vi "CRYPlot Intensity Graph.vi"(6 "Graph Set?":bool, 7 "pGraph VI In":refnum<vi>, 9 "Flattened Intensity Property":string, 11 "Selected Rows In":i32[](array[numeric])) -> (0 "ItemSyms":i32[](array[numeric]), 1 "Color Info":u32[](array[numeric]), 2 "Wave Names":string[](array[string]), 3 "All Rows Out":i32[](array[numeric]))   [LabVIEW 2013]
uses:
  <vilib>/Analysis/4window.llb/windowTd.ctl
  CRYWindow/DataView/Control/CRYIntensity Property.ctl
  <vilib>/Analysis/NI_AALPro.lvlib
panel:
  in  "Intensity Property":T1 {"Type" items=["Rectangle"=0, "Hanning"=1, "Hamming"=2, "Blackman-Harris"=3, "Exact Blackman"=4, "Blackman"=5, "Flat Top"=6, "4 Term B-Harris"=7, "7 Term B-Harris"=8, "Low Sidelobe"=9, "Blackman Nuttall"=11, "Triangle"=30, "Bartlett-Hanning"=31, "Bohman"=32, "Parzen"=33, "Welch"=34, "Kaiser"=60, "Dolph-Chebyshev"=61, "Gaussian"=62]}
  in  "32 ice":u32[](array[numeric])=[2155776, 2155776, 2155776, 2155776, 2155776, 2155776, 2155776, 2155776, 127491, 127491, 127491, 127491, 127491, 127491, 127491, 127491, 522752, 522752, 522752, 522752, 522752, 522752, 522752, 522752, 64018, 64018, 64018, 64018, 64018, 64018, 64018, 64018, 63778, 63778, 63778, 63778, 63778, 63778, 63778, 63778, 63790, 63790, 63790, 63790, 63790, 63790, 63790, 63790, 63797, 63797, 63797, 63797, 63797, 63797, 63797, 63797, 63807, 63807, 63807, 63807, 63807, 63807, 63807, 63807, 64068, 64068, 64068, 64068, 64068, 64068, 64068, 64068, 63828, 63828, 63828, 63828, 63828, 63828, 63828, 63828, 63833, 63833, 63833, 63833, 63833, 63833, 63833, 63833, 63836, 63836, 63836, 63836, 63836, 63836, 63836, 63836, 63836, 63836, 63836, 63836, 63836, 63836, 63836, 63836, 61790, 61790, 61790, 61790, 61790, 61790, 61790, 61790, 58464, 58464, 58464, 58464, 58464, 58464, 58464, 58464, 55387, 55387, 55387, 55387, 55387, 55387, 55387, 55387, 51286, 51286, 51286, 51286, 51286, 51286, 51286, 51286, 47440, 47440, 47440, 47440, 47440, 47440, 47440, 47440, 40284, 40284, 40284, 40284, 40284, 40284, 40284, 40284, 34154, 34154, 34154, 34154, 34154, 34154, 34154, 34154, 28540, 28540, 28540, 28540, 28540, 28540, 28540, 28540, 20113, 20113, 20113, 20113, 20113, 20113, 20113, 20113, 12193, 12193, 12193, 12193, 12193, 12193, 12193, 12193, 12714, 12714, 12714, 12714, 12714, 12714, 12714, 12714, 7351, 7351, 7351, 7351, 7351, 7351, 7351, 7351, 4800, 4800, 4800, 4800, 4800, 4800, 4800, 4800, 195, 195, 195, 195, 195, 195, 195, 195, 189, 189, 189, 189, 189, 189, 189, 189, 183, 183, 183, 183, 183, 183, 183, 183, 175, 175, 175, 175, 175, 175, 175, 175, 164, 164, 164, 164, 164, 164, 164, 164, 155, 155, 155, 155, 155, 155, 155, 155]
  in  "32 colour":u32[](array[numeric])=[2161664, 2161664, 2161664, 2161664, 2161664, 2161664, 2161664, 2161664, 588800, 588800, 588800, 588800, 588800, 588800, 588800, 588800, 523264, 523264, 523264, 523264, 523264, 523264, 523264, 523264, 64512, 64512, 64512, 64512, 64512, 64512, 64512, 64512, 64512, 64512, 64512, 64512, 64512, 64512, 64512, 64512, 64512, 64512, 64512, 64512, 64512, 64512, 64512, 64512, 64512, 64512, 64512, 64512, 64512, 64512, 64512, 64512, 64512, 64512, 64512, 64512, 64512, 64512, 64512, 64512, 64512, 64512, 64512, 64512, 64512, 64512, 64512, 64512, 64512, 64512, 64512, 64512, 64512, 64512, 64512, 64512, 64512, 64512, 64512, 64512, 64512, 64512, 64512, 64512, 64512, 64512, 64512, 64512, 64512, 64512, 64512, 64512, 64512, 64512, 64512, 64512, 64512, 64512, 64512, 64512, 64512, 64512, 64512, 64512, 64512, 64512, 64512, 64512, 64512, 64512, 64512, 64512, 64512, 64512, 64512, 64512, 64512, 64512, 64512, 64512, 64512, 64512, 64512, 64512, 64525, 64525, 64525, 64525, 64525, 64525, 64525, 64525, 64541, 64541, 64541, 64541, 64541, 64541, 64541, 64541, 64557, 64557, 64557, 64557, 64557, 64557, 64557, 64557, 64573, 64573, 64573, 64573, 64573, 64573, 64573, 64573, 64333, 64333, 64333, 64333, 64333, 64333, 64333, 64333, 64349, 64349, 64349, 64349, 64349, 64349, 64349, 64349, 64621, 64621, 64621, 64621, 64621, 64621, 64621, 64621, 64636, 64636, 64636, 64636, 64636, 64636, 64636, 64636, 64653, 64653, 64653, 64653, 64653, 64653, 64653, 64653, 64670, 64670, 64670, 64670, 64670, 64670, 64670, 64670, 64685, 64685, 64685, 64685, 64685, 64685, 64685, 64685, 64701, 64701, 64701, 64701, 64701, 64701, 64701, 64701, 64717, 64717, 64717, 64717, 64717, 64717, 64717, 64717, 64733, 64733, 64733, 64733, 64733, 64733, 64733, 64733, 64749, 64749, 64749, 64749, 64749, 64749, 64749, 64749, 64764, 64764, 64764, 64764, 64764, 64764, 64764, 64764]
  in  "256 log down":u32[](array[numeric])=[16777215, 14737632, 13487565, 12632256, 11908533, 11382189, 10921638, 10526880, 10132122, 9803157, 9539985, 9276813, 9013641, 8816262, 8553090, 8421504, 8224125, 8026746, 7895160, 7697781, 7566195, 7434609, 7303023, 7171437, 7039851, 6908265, 6776679, 6710886, 6579300, 6447714, 6381921, 6316128, 6184542, 6118749, 5987163, 5921370, 5855577, 5789784, 5658198, 5592405, 5526612, 5460819, 5395026, 5329233, 5263440, 5197647, 5131854, 5066061, 5000268, 4934475, 4868682, 4802889, 4737096, 4671303, 4605510, 4605510, 4539717, 4473924, 4408131, 4342338, 4342338, 4276545, 4210752, 4210752, 4144959, 4079166, 4013373, 4013373, 3947580, 3881787, 3881787, 3815994, 3750201, 3750201, 3684408, 3684408, 3618615, 3552822, 3552822, 3487029, 3487029, 3421236, 3421236, 3355443, 3289650, 3289650, 3223857, 3223857, 3158064, 3158064, 3092271, 3092271, 3026478, 3026478, 2960685, 2960685, 2894892, 2894892, 2829099, 2829099, 2763306, 2763306, 2763306, 2697513, 2697513, 2631720, 2631720, 2565927, 2565927, 2500134, 2500134, 2500134, 2434341, 2434341, 2368548, 2368548, 2368548, 2302755, 2302755, 2236962, 2236962, 2236962, 2171169, 2171169, 2171169, 2105376, 2105376, 2105376, 2039583, 2039583, 1973790, 1973790, 1973790, 1907997, 1907997, 1907997, 1842204, 1842204, 1842204, 1776411, 1776411, 1776411, 1710618, 1710618, 1710618, 1644825, 1644825, 1644825, 1579032, 1579032, 1579032, 1579032, 1513239, 1513239, 1513239, 1447446, 1447446, 1447446, 1381653, 1381653, 1381653, 1381653, 1315860, 1315860, 1315860, 1315860, 1250067, 1250067, 1250067, 1184274, 1184274, 1184274, 1184274, 1118481, 1118481, 1118481, 1118481, 1052688, 1052688, 1052688, 1052688, 986895, 986895, 986895, 921102, 921102, 921102, 921102, 921102, 855309, 855309, 855309, 855309, 789516, 789516, 789516, 789516, 723723, 723723, 723723, 723723, 657930, 657930, 657930, 657930, 657930, 592137, 592137, 592137, 592137, 526344, 526344, 526344, 526344, 526344, 460551, 460551, 460551, 460551, 460551, 394758, 394758, 394758, 394758, 328965, 328965, 328965, 328965, 328965, 263172, 263172, 263172, 263172, 263172, 197379, 197379, 197379, 197379, 197379, 131586, 131586, 131586, 131586, 131586, 131586, 65793, 65793, 65793, 65793, 65793, 0, 0, 0, 0, 0, 0]
  in  "256 log up":u32[](array[numeric])=[16777215, 16777215, 16777215, 16777215, 16777215, 16777215, 16711422, 16711422, 16711422, 16711422, 16711422, 16645629, 16645629, 16645629, 16645629, 16645629, 16645629, 16579836, 16579836, 16579836, 16579836, 16579836, 16514043, 16514043, 16514043, 16514043, 16514043, 16448250, 16448250, 16448250, 16448250, 16448250, 16316664, 16382457, 16382457, 16382457, 16382457, 16316664, 16316664, 16316664, 16316664, 16250871, 16250871, 16250871, 16250871, 16250871, 16185078, 16185078, 16185078, 16185078, 16119285, 16119285, 16119285, 16119285, 16119285, 16053492, 16053492, 16053492, 16053492, 15987699, 15987699, 15987699, 15987699, 15921906, 15987699, 15921906, 15921906, 15856113, 15856113, 15856113, 15856113, 15856113, 15790320, 15790320, 15790320, 15724527, 15724527, 15724527, 15724527, 15658734, 15658734, 15658734, 15658734, 15592941, 15592941, 15592941, 15592941, 15527148, 15527148, 15527148, 15461355, 15461355, 15461355, 15461355, 15395562, 15395562, 15395562, 15395562, 15329769, 15329769, 15329769, 15263976, 15263976, 15263976, 15198183, 15198183, 15198183, 15198183, 15132390, 15132390, 15132390, 15066597, 15066597, 15066597, 15000804, 15000804, 15000804, 14935011, 14935011, 14935011, 14869218, 14869218, 14869218, 14803425, 14803425, 14803425, 14737632, 14737632, 14671839, 14671839, 14671839, 14606046, 14606046, 14606046, 14540253, 14540253, 14540253, 14474460, 14474460, 14408667, 14408667, 14408667, 14342874, 14342874, 14277081, 14277081, 14277081, 14211288, 14211288, 14145495, 14145495, 14079702, 14079702, 14013909, 14013909, 14013909, 13948116, 13948116, 13882323, 13882323, 13816530, 13816530, 13750737, 13750737, 13684944, 13684944, 13619151, 13619151, 13553358, 13553358, 13487565, 13487565, 13421772, 13421772, 13355979, 13290186, 13290186, 13224393, 13224393, 13158600, 13092807, 13092807, 13027014, 13027014, 12961221, 12895428, 12895428, 12829635, 12763842, 12763842, 12698049, 12632256, 12566463, 12566463, 12500670, 12434877, 12434877, 12369084, 12303291, 12237498, 12171705, 12171705, 12105912, 12040119, 11974326, 11908533, 11842740, 11776947, 11711154, 11645361, 11579568, 11513775, 11447982, 11382189, 11316396, 11250603, 11184810, 11119017, 10987431, 10921638, 10855845, 10790052, 10658466, 10592673, 10461087, 10395294, 10329501, 10197915, 10066329, 10000536, 9868950, 9737364, 9605778, 9474192, 9342606, 9211020, 9079434, 8882055, 8750469, 8553090, 8421504, 8224125, 7960953, 7763574, 7500402, 7237230, 6974058, 6645093, 6316128, 5855577, 5395026, 4868682, 4210752, 3289650, 2105376, 0]
  in  "256 fire":u32[](array[numeric])=[16777215, 16777215, 16777215, 16777215, 16777215, 16777215, 16777215, 16777215, 16777212, 16777209, 16777205, 16777202, 16777199, 16777196, 16777193, 16777190, 16777186, 16777183, 16777180, 16777177, 16777174, 16777170, 16777167, 16777164, 16777161, 16777158, 16777154, 16777151, 16777148, 16777145, 16777142, 16777139, 16777135, 16777132, 16777129, 16777126, 16777123, 16777119, 16777116, 16777113, 16777110, 16777107, 16777103, 16777100, 16777097, 16777094, 16777091, 16777088, 16777084, 16777081, 16777078, 16777075, 16777072, 16777068, 16777065, 16777062, 16777059, 16777056, 16777052, 16777049, 16777046, 16777043, 16777040, 16777037, 16777033, 16777030, 16777027, 16777024, 16777021, 16777017, 16777014, 16777011, 16777008, 16777005, 16777001, 16776998, 16776995, 16776992, 16776989, 16776986, 16776982, 16776979, 16776976, 16776973, 16776970, 16776966, 16776963, 16776960, 16776192, 16775424, 16774400, 16773632, 16772864, 16772096, 16771328, 16770560, 16769536, 16768768, 16768000, 16767232, 16766464, 16765440, 16764672, 16763904, 16763136, 16762368, 16761344, 16760576, 16759808, 16759040, 16758272, 16757504, 16756480, 16755712, 16754944, 16754176, 16753408, 16752384, 16751616, 16750848, 16750080, 16749312, 16748288, 16747520, 16746752, 16745984, 16745216, 16744448, 16743424, 16742656, 16741888, 16741120, 16740352, 16739328, 16738560, 16737792, 16737024, 16736256, 16735232, 16734464, 16733696, 16732928, 16732160, 16731392, 16730368, 16729600, 16728832, 16728064, 16727296, 16726272, 16725504, 16724736, 16723968, 16723200, 16722176, 16721408, 16720640, 16719872, 16719104, 16718336, 16717312, 16716544, 16715776, 16715008, 16714240, 16713216, 16712448, 16711680, 16515072, 16318464, 16056320, 15859712, 15663104, 15466496, 15269888, 15073280, 14811136, 14614528, 14417920, 14221312, 14024704, 13762560, 13565952, 13369344, 13172736, 12976128, 12713984, 12517376, 12320768, 12124160, 11927552, 11730944, 11468800, 11272192, 11075584, 10878976, 10682368, 10420224, 10223616, 10027008, 9830400, 9633792, 9371648, 9175040, 8978432, 8781824, 8585216, 8388608, 8126464, 7929856, 7733248, 7536640, 7340032, 7077888, 6881280, 6684672, 6488064, 6291456, 6029312, 5832704, 5636096, 5439488, 5242880, 5046272, 4784128, 4587520, 4390912, 4194304, 3997696, 3735552, 3538944, 3342336, 3145728, 2949120, 2686976, 2490368, 2293760, 2097152, 1900544, 1703936, 1441792, 1245184, 1048576, 851968, 655360, 393216, 196608, 65793, 65793, 65793, 65793, 65793, 65793, 65793, 65793, 0]
  in  "window info":cluster{"type":T2, "length":i32}={"type"=1, "length"=64} {"type" items=["Rectangle"=0, "Hanning"=1, "Hamming"=2, "Blackman-Harris"=3, "Exact Blackman"=4, "Blackman"=5, "Flat Top"=6, "4 Term B-Harris "=7, "7 Term B-Harris"=8, "Low Sidelobe"=9, "Blackman Nuttall"=11, "Triangle"=30, "Bartlett-Hanning"=31, "Bohman"=32, "Parzen"=33, "Welch"=34, "Kaiser"=60, "Dolph-Chebyshev"=61, "Gaussian"=62]}
  in  "time-freq sampling info":cluster{"time steps":i32, "frequency bins":i32}={"time steps"=512, "frequency bins"=1024}
  in  "256 rainbow":u32[](array[numeric])=[16777215, 8126719, 7864574, 7536895, 7274750, 6947071, 6684926, 6357247, 6095102, 5767423, 5505278, 5177599, 4915454, 4587775, 4325630, 3997951, 3735806, 3408127, 3145982, 2818303, 2556158, 2228479, 1966334, 1638655, 1376510, 1048831, 786686, 459007, 196862, 767, 1790, 3071, 4094, 5375, 6398, 7679, 8702, 9983, 11006, 12287, 13310, 14591, 15614, 16895, 17918, 19199, 20222, 21503, 22526, 23807, 24830, 26111, 27134, 28415, 29438, 30719, 31486, 33023, 33790, 35327, 36094, 37631, 38398, 39935, 40702, 42239, 43006, 44543, 45310, 46847, 47614, 49151, 49918, 51455, 52222, 53759, 54526, 56063, 56830, 58367, 59134, 60671, 61694, 62975, 63998, 65279, 65274, 65527, 65265, 65518, 65256, 65509, 65247, 65500, 65238, 65491, 65229, 65482, 65220, 65473, 65211, 65464, 65202, 65455, 65193, 65446, 65184, 65437, 65175, 65428, 65166, 65419, 65157, 65410, 65149, 65401, 65140, 65392, 65131, 65383, 65122, 65374, 65113, 65365, 65104, 65356, 65095, 65347, 65086, 65338, 65077, 65329, 65068, 65320, 65059, 65311, 65050, 65302, 65041, 65293, 65032, 65284, 130560, 392960, 720384, 982784, 1310208, 1572608, 1900032, 2162432, 2489856, 2752256, 3079680, 3342080, 3669504, 3931904, 4259328, 4521728, 4849152, 5111552, 5438976, 5701376, 6028800, 6291200, 6618624, 6881024, 7208448, 7470848, 7798272, 8126208, 8322560, 8716032, 8912384, 9305856, 9502208, 9895680, 10092032, 10485504, 10681856, 11075328, 11271680, 11665152, 11861504, 12254976, 12451328, 12844800, 13041152, 13434624, 13630976, 14024448, 14220800, 14614272, 14810624, 15204096, 15400448, 15793920, 15990272, 16383744, 16580096, 16776192, 16709376, 16773888, 16707072, 16771584, 16704768, 16769280, 16702464, 16766976, 16700160, 16764672, 16697856, 16762368, 16695552, 16760064, 16693248, 16757760, 16690944, 16755456, 16688640, 16753152, 16686336, 16750848, 16684032, 16748544, 16681728, 16746240, 16679680, 16743936, 16677376, 16741632, 16675072, 16739328, 16672768, 16737024, 16670464, 16734720, 16668160, 16732416, 16665856, 16730112, 16663552, 16727808, 16661248, 16725504, 16658944, 16723200, 16656640, 16720896, 16654336, 16718592, 16652032, 16716288, 16649728, 16713984, 16712960, 0]
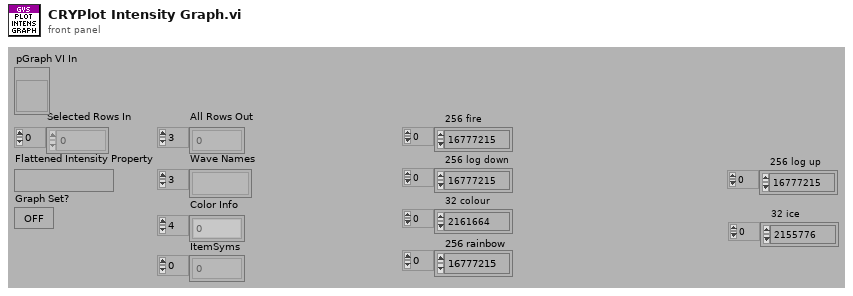
[diagram p1: front panel]
types:
  T1 = typedef "CRYIntensity Property.ctl" = cluster{"Time Steps":i32, "Frequency Bins":i32, "Type":u32, "Length":i32, "Map Type":enum16{"fire", "rainbow", "grey", "inverse grey", "ice", "original"}}
  T2 = typedef "NI_AALPro.lvlib/windowTd.ctl" = u32
  T3 = typedef "CRYWaveform Cluster.ctl" = cluster{"Waveform":cluster{"X0":dbl, "dX":dbl, "Y":sgl[]}, "X data":u16, "Y data":u16, "Y axis":u16, "X unit":string, "Y unit":string, "Y dB ref":dbl, "display Y":bool, "display X":bool, "Overload?":bool, "Test Info":string, "Step No.":i32, "Name":string, "protected":bool, "Sqc history":string[], "Signal Channel ID":i32, "Plot Settings":cluster{"Color":u32, "Interpolation":u8, "Point Style":u8, "Line Style":u8, "Point Color":u32, "Line Width":u8, "Bar Plot Style":u8, "Fill To":i16}, "AutoProtect":bool}
  T4 = enum16{"OK", "Yes", "YesNo", "YesNoCancel", "ReplaceAppend"}
  T5 = typedef "CRYStimulus Test Infor Cluster.ctl" = cluster{"Stimulus Type":string, "Signal Type":string, "In/Out":bool, "FAPS":cluster{"freq":dbl, "ampl":dbl, "cycles":dbl, "samples":i32}[], "Sampling Rate":dbl, "Samples":i32, "Analysis Param":string, "Resolution":u16, "Steps":u32, "Analysis Value":dbl[], "Diff Freq":dbl, "FStart":dbl, "FStop":dbl, "Calibration Param":string, "Anti Alias":dbl, "Level Out1":dbl, "Level Out2":dbl, "EQ":bool}
  T6 = enum16{"fire", "rainbow", "grey", "inverse grey", "ice", "original"}
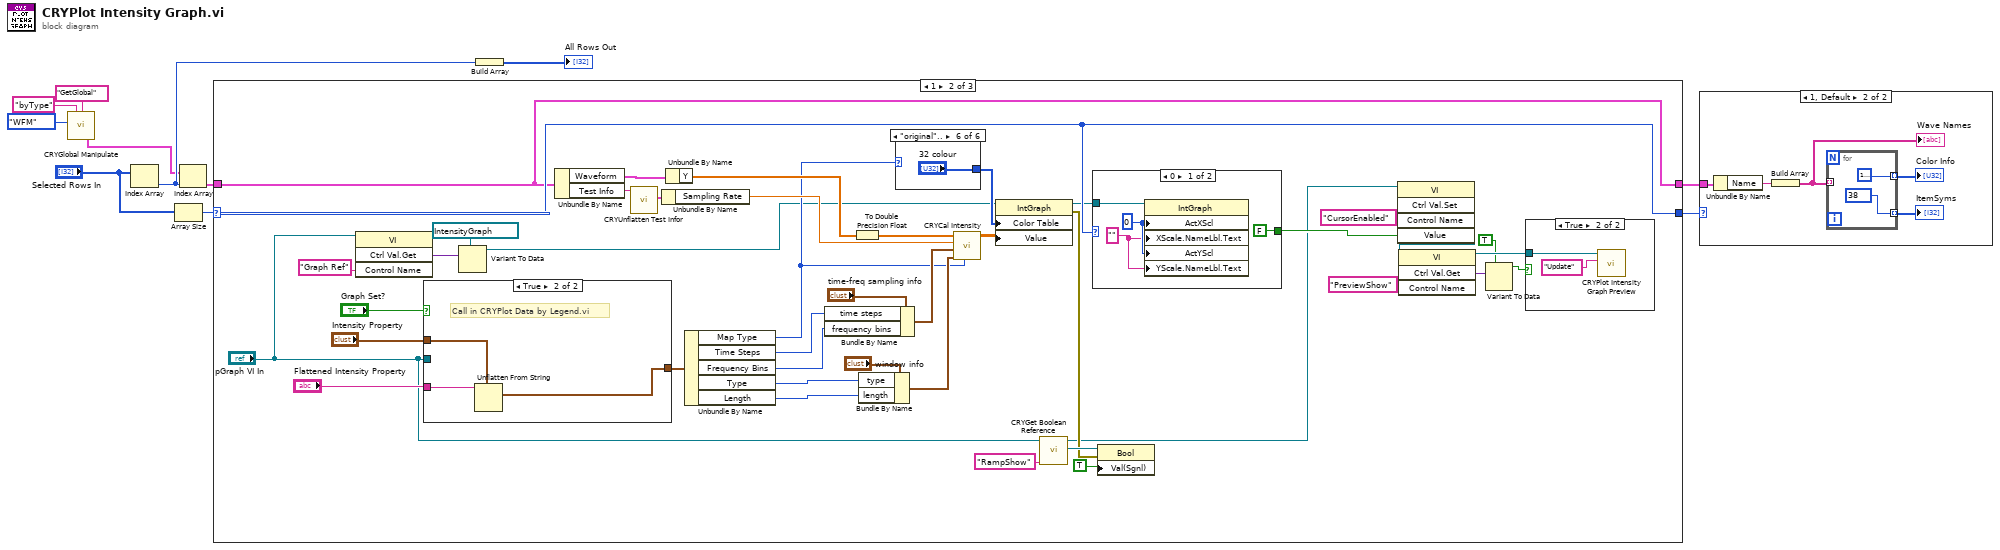
[diagram p0: block diagram]
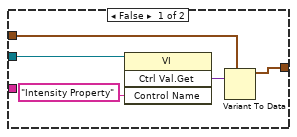
[diagram p4: hidden frame]
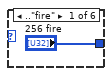
[diagram p5: hidden frame]
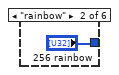
[diagram p6: hidden frame]
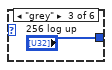
[diagram p7: hidden frame]
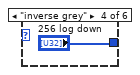
[diagram p8: hidden frame]
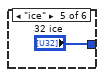
[diagram p9: hidden frame]
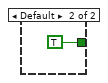
[diagram p11: hidden frame]
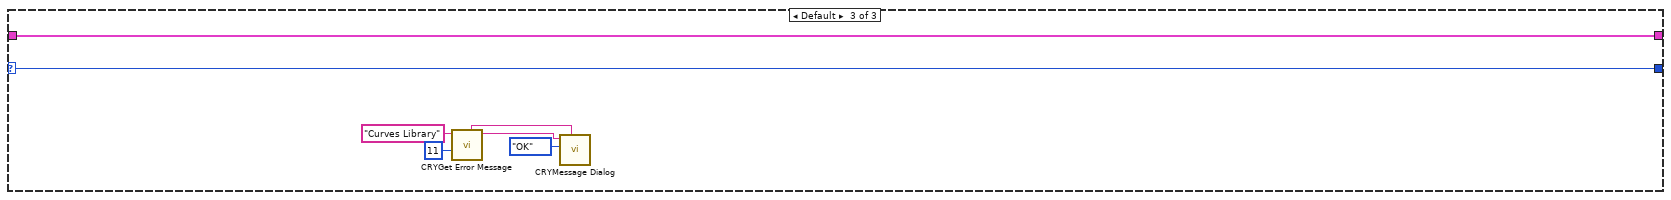
[diagram p12: hidden frame]
diagram:
  n1 = call "CRYGlobal Manipulate.vi"("Type"=enum16{"Curves", "Values", "Results", "WFM"}."WFM", "sOption"="byType", "sAction"="GetGlobal") -> ("WFM Out"=w1:T3[])  [unwired: 6 in, 6 out]
  n2 = Index Array(array="Selected Rows In") -> (element=w6:i32)  [unwired: 1 in]
  n3 = Array Size(array="Selected Rows In") -> (size(s)=w9:i32)
  n4 = Index Array(array=w1, index=w6) -> (element=w10:T3)
  n5 = case shown="1" w9 {
    selector: w9 -> [w13 w44 w83]
    tunnel: w10 -> [w12 w43 w82]
    tunnel: [w13 w44 w83] -> w8
    tunnel: [w12 w43 w82] -> w7
    frame 0 {
    }
    frame 1 {
      n6 = invoke class="VI" method="Ctrl Val.Get"(reference="pGraph VI In", "Control Name"="Graph Ref") -> ("Get Control Value Variant"=w16:variant)  [unwired: 2 in, 3 out]
      n7 = case shown="True" "Graph Set?" {
        tunnel: [w60 w61] -> w26
        tunnel: "Intensity Property" -> [w59 w62]
        tunnel: "pGraph VI In" -> [w58 _]
        tunnel: "Flattened Intensity Property" -> [_ w63]
        frame False {
          n8 = invoke class="VI" method="Ctrl Val.Get"(reference=w58, "Control Name"="Intensity Property") -> ("Get Control Value Variant"=w56:variant)  [unwired: 2 in, 3 out]
          n9 = Variant To Data(type=w59, Variant=w56) -> (data=w60:T1)  [unwired: 1 in, 1 out]
        }
        frame True {
          # "Call in CRYPlot Data by Legend.vi"
          n10 = Unflatten From String(type=w62, binary string=w63) -> (value=w61:T1)  [unwired: 3 in, 2 out]
        }
      }
      n11 = Variant To Data(type=refnum<vi> refnum ("Graph Ref"), Variant=w16) -> (data=w15:refnum<vi>)  [unwired: 1 in, 1 out]
      n12 = Unbundle By Name(w43) -> ("Waveform"=w46:cluster{"X0":dbl, "dX":dbl, "Y":sgl[]}, "Test Info"=w45:string)
      n13 = call "CRYUnflatten Test Infor.vi"("Falattend test infor"=w45) -> ("unflattened test infor data"=w55:T5)  [unwired: 8 in, 1 out]
      n14 = Unbundle By Name(w55) -> ("Sampling Rate"=w41:dbl)
      n15 = Unbundle By Name(w46) -> ("Y"=w42:sgl[])
      n16 = Unbundle By Name(w26) -> ("Map Type"=w24:T6, "Time Steps"=w31:i32, "Frequency Bins"=w30:i32, "Type"=w35:u32, "Length"=w34:i32)
      n17 = Bundle By Name(cluster="time-freq sampling info", "time steps"=w31, "frequency bins"=w30) -> (w33:cluster{"time steps":i32, "frequency bins":i32})
      n18 = To Double Precision Float(number=w42) -> (double precision float=w39:dbl[])
      n19 = Bundle By Name(cluster="window info", "type"=w35, "length"=w34) -> (w32:cluster{"type":T2, "length":i32})
      n20 = case shown="\"original\".." w24 {
        tunnel: ["256 fire" "256 rainbow" "256 log up" "256 log down" "32 ice" "32 colour"] -> w36
        frame .."fire" {
        }
        frame "rainbow" {
        }
        frame "grey" {
        }
        frame "inverse grey" {
        }
        frame "ice" {
        }
        frame "original".. {
        }
      }
      n21 = call "CRYCal Intensity.vi"("map selector"=w24, "window info"=w32, "time-freq sampling info"=w33, "Fs"=w41, "Y"=w39) -> ("STFT Spectrum"=w40:dbl[][])  [unwired: 6 in]
      n22 = property class="IntGraph"(reference=w15, "Color Table"=w36, "Value"=w40) -> (reference out=w25:refnum<vi>, error out=w20:errorcluster)  [unwired: 1 in]
      n23 = call "CRYGet Boolean Reference.vi"("Label Name"="RampShow", "VI Refnum"="pGraph VI In") -> ("Boolean Ref"=w22:refnum<vi>, "VI Refnum Out"=w14:refnum<vi>)  [unwired: 7 in, 1 out]
      n24 = case shown="0" w44 {
        tunnel: w25 -> [w73 _]
        tunnel: [FALSE TRUE] -> w53
        frame 0 {
          w75 = 0 ("Active X Scale")
          w74 = "" ("X Scale.Name Label.Text")
          n25 = property class="IntGraph"(reference=w73, "ActXScl"=w75, "XScale.NameLbl.Text"=w74, "ActYScl"=w75, "YScale.NameLbl.Text"=w74) -> ()  [unwired: 1 in, 2 out]
        }
        frame Default {
        }
      }
      n26 = property class="Bool"(reference=w22, error in=w20, "Val(Sgnl)"=TRUE) -> ()  [unwired: 2 out]
      n27 = invoke class="VI" method="Ctrl Val.Set"(reference=w14, "Control Name"="CursorEnabled", "Value"=w53) -> (reference out=w51:refnum<vi>)  [unwired: 2 in, 4 out]
      n28 = invoke class="VI" method="Ctrl Val.Get"(reference=w51, "Control Name"="PreviewShow") -> (reference out=w50:refnum<vi>, "Get Control Value Variant"=w49:variant)  [unwired: 2 in, 2 out]
      n29 = Variant To Data(type=TRUE, Variant=w49) -> (data=w47:bool)  [unwired: 1 in, 1 out]
      n30 = case shown="True" w47 {
        tunnel: w50 -> [_ w71]
        frame False {
        }
        frame True {
          n31 = call "CRYPlot Intensity Graph Preview.vi"("sOption"="Update", "IntensityGraph VI Ref"=w71) -> ()  [unwired: 10 in]
        }
      }
    }
    frame Default {
      n32 = call "CRYGet Error Message.vi"("Error No"=11, "Kind"="Curves Library") -> ("Message"=w77:string, "Window Title"=w78:string)  [unwired: 4 in, 4 out]
      n33 = call "CRYMessage Dialog.vi"("Window Title"=w78, "YesNoCancel"=T4."OK", "Message Content"=w77) -> ()  [unwired: 7 in, 2 out]
    }
  }
  n34 = Build Array(w6) -> (→"All Rows Out":i32[])
  n35 = case shown="1, Default" w8 {
    tunnel: w7 -> [_ w84]
    frame 0 {
    }
    frame 1, Default {
      n36 = Unbundle By Name(w84) -> ("Name"=w88:string)
      n37 = Build Array(w88) -> (w87:string[])
      "Wave Names" <- w87
      n38 = for {
        tunnel: w87 -> [_] mode=indexing
        tunnel: [u32 16777226] -> w86 mode=indexing
        tunnel: [38] -> w85 mode=indexing
      }
      "Color Info" <- w86
      "ItemSyms" <- w85
    }
  }
